vi "go to last element.vi"(8 "error in (no error)":errorcluster, 11 "Array in":refnum<vi>) -> (0 "error out":errorcluster, 3 "reference out":refnum<vi>)   [LabVIEW 2014, in "Tagbus PID Module editor node.lvclass"]
uses:
  Tagbus PID Module editor node.lvclass
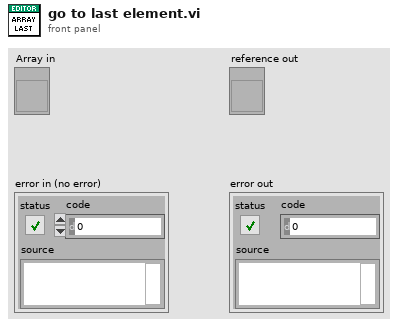
[diagram p1: front panel]
types:
  T1 = cluster{"Loop ID":string, "Tags":cluster{"Setpoint":string, "Process Variable":string, "Output":string}, "Gains":cluster{"P":dbl, "I":dbl, "D":dbl}, "Range":cluster{"High":dbl, "Low":dbl}}[]
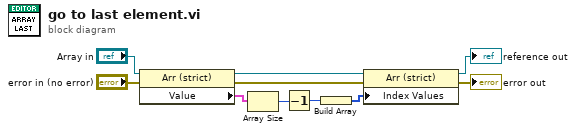
[diagram p0: block diagram]
diagram:
  n1 = property class="Arr (strict)"(reference="Array in", error in="error in (no error)") -> (reference out=w6:refnum<vi>, error out=w3:errorcluster, "Value"=w9:T1)
  n2 = Array Size(array=w9) -> (size(s)=w10:i32)
  n3 = Decrement(x=w10) -> (x-1=w8:i32)
  n4 = Build Array(w8) -> (w7:i32[])
  n5 = property class="Arr (strict)"(reference=w6, error in=w3, "Index Values"=w7) -> (reference out=→"reference out":refnum<vi>, error out=→"error out":errorcluster)
